vi "Message En-Q.vi"(7 "Priority Message":bool, 8 "error in":errorcluster, 11 "Message Q Type":T1) -> (0 "error out":errorcluster)   [LabVIEW 2020, in "Hardware.lvlib"]
doc: "ENqueue a message for this component."
uses:
  Hardware.lvlib
  Message Type.ctl
  Message FGV Actions.ctl
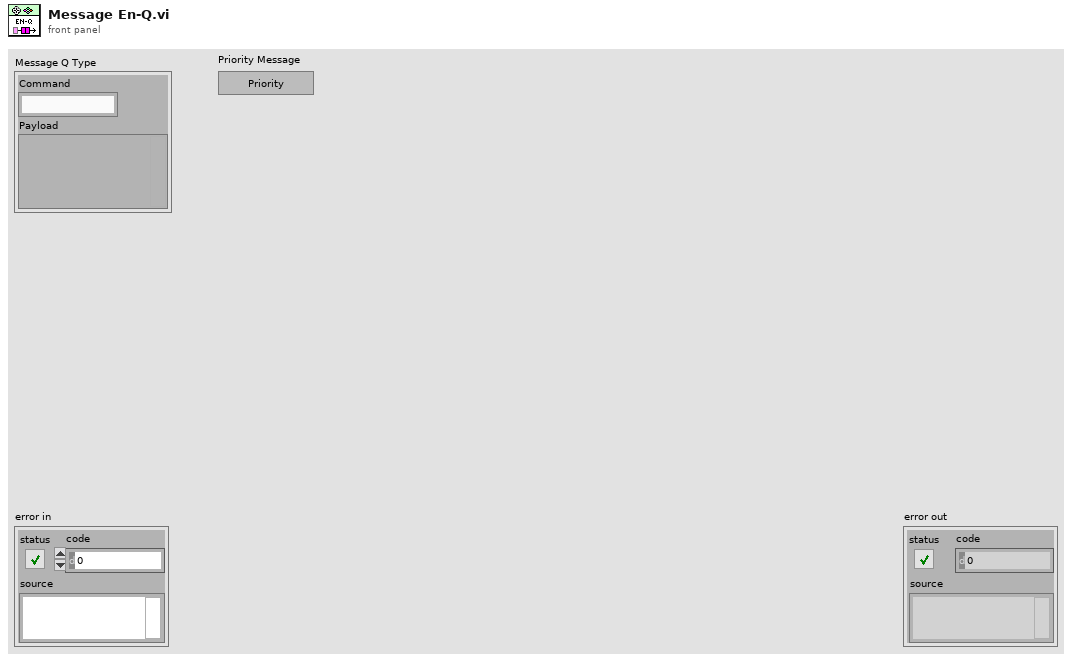
[diagram p1: front panel]
types:
  T1 = typedef "Hardware.lvlib/Message Type.ctl" = cluster{"Command":string, "Payload":variant}
  T2 = typedef "Hardware.lvlib/Message FGV Actions.ctl" = enum16{"Get", "Obtain", "Release", "Flush"}
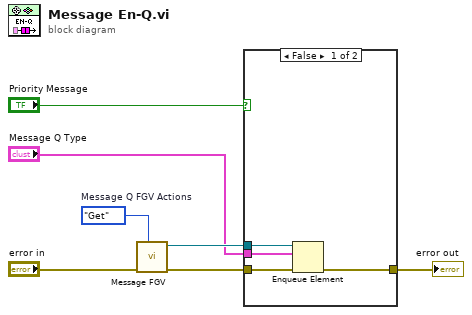
[diagram p0: block diagram]
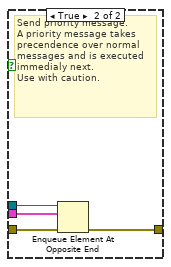
[diagram p2: hidden frame]
diagram:
  w5 = Message_FGV_Actions."Get"  # Message Q FGV Actions
  n1 = call "Message FGV.vi"("Message Q FGV Actions"=w5, "error in"="error in") -> ("error out"=w6:errorcluster, "queue ref out"=w3:refnum<queue>)  [unwired: 6 in, 2 out]
  n2 = case shown="False" "Priority Message" {
    tunnel: w6 -> [w11 w15]
    tunnel: [w10 w14] -> w4
    tunnel: w3 -> [w9 w13]
    tunnel: "Message Q Type" -> [w8 w12]
    frame False {
      n3 = Enqueue Element(queue=w9, element=w8, error in (no error)=w11) -> (error out=w10:errorcluster)  [unwired: 1 in, 2 out]
    }
    frame True {
      # "Send priority message.\nA priority message takes precendence over normal messages and is executed immedialy next.\nUse with caution."
      n4 = Enqueue Element At Opposite End(queue=w13, element=w12, error in (no error)=w15) -> (error out=w14:errorcluster)  [unwired: 1 in, 2 out]
    }
  }
  "error out" <- w4
